vi "svx_Add SVTWav Info.vi"(6 "SVT WAV info":T1, 8 "error in (no error)":errorcluster, 11 "wave file path in":path) -> (0 "error out":errorcluster, 3 "wave file path":path)   [LabVIEW 2017]
uses:
  <vilib>/addons/_NISVFA/_Shared subVIs/Controls/SVT WAV Info.ctl
  <vilib>/addons/_NISVFA/_Shared subVIs/Controls/DAQ Coupling for SVT WAV Info.ctl
  <vilib>/addons/_NISVFA/_Shared subVIs/Controls/DAQ Polarity for SVT WAV Info.ctl
  <vilib>/addons/_NISVFA/_Shared subVIs/Controls/DAQ Terminal Configuration for SVT WAV Info.ctl
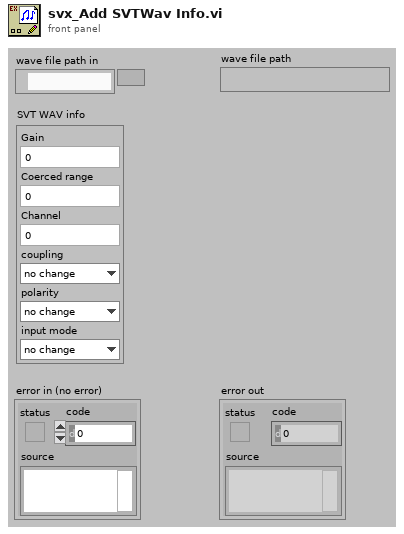
[diagram p1: front panel]
types:
  T1 = typedef "SVT WAV Info.ctl" = cluster{"Gain":u16, "Coerced range":u16, "Channel":u16, "coupling":T2, "polarity":T3, "input mode":T4}
  T2 = typedef "DAQ Coupling for SVT WAV Info.ctl" = enum16{"no change", "DC", "AC", "ground", "internal reference"}
  T3 = typedef "DAQ Polarity for SVT WAV Info.ctl" = enum16{"no change", "bipolar", "unipolar"}
  T4 = typedef "DAQ Terminal Configuration for SVT WAV Info.ctl" = enum16{"no change", "differential", "rse", "nrse", "pseudodifferential"}
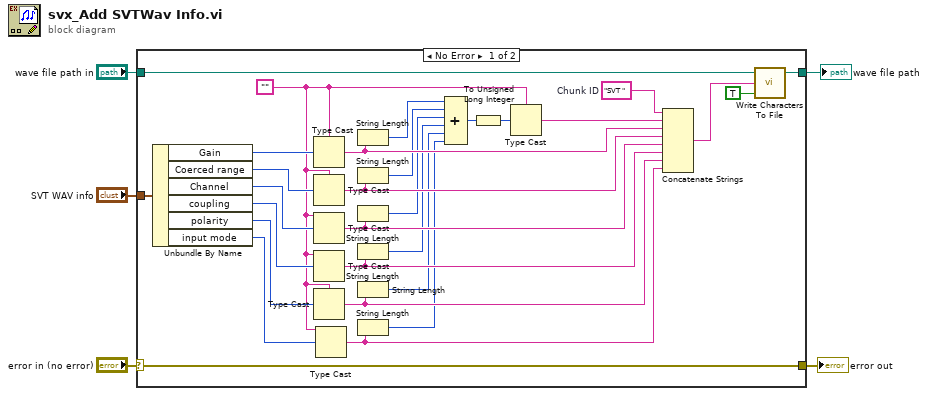
[diagram p0: block diagram]
diagram:
  n1 = case shown="No Error" "error in (no error)" {
    selector: "error in (no error)" -> [w11 w36]
    tunnel: [w11 w36] -> w4
    tunnel: "wave file path in" -> [w10 w35]
    tunnel: "SVT WAV info" -> [w9 _]
    tunnel: [w8 w35] -> w1
    frame No Error {
      w33 = "SVT "  # Chunk ID
      w12 = ""
      n2 = Unbundle By Name(w9) -> ("Gain"=w30:u16, "Coerced range"=w27:u16, "Channel"=w26:u16, "coupling"=w25:T2, "polarity"=w24:T3, "input mode"=w7:T4)
      n3 = Type Cast(type=w12, x=w30) -> (*(type *) &x=w31:string)
      n4 = Type Cast(type=w12, x=w27) -> (*(type *) &x=w23:string)
      n5 = Type Cast(type=w12, x=w26) -> (*(type *) &x=w22:string)
      n6 = Type Cast(type=w12, x=w25) -> (*(type *) &x=w21:string)
      n7 = Type Cast(type=w12, x=w24) -> (*(type *) &x=w20:string)
      n8 = Type Cast(type=w12, x=w7) -> (*(type *) &x=w6:string)
      n9 = String Length(string=w31) -> (length=w19:i32)
      n10 = String Length(string=w23) -> (length=w18:i32)
      n11 = String Length(string=w22) -> (length=w17:i32)
      n12 = String Length(string=w21) -> (length=w16:i32)
      n13 = String Length(string=w20) -> (length=w15:i32)
      n14 = String Length(string=w6) -> (length=w13:i32)
      n15 = Compound Arithmetic op=ADD(w19, w18, w17, w16, w15, w13) -> (w14:i32)
      n16 = To Unsigned Long Integer(number=w14) -> (unsigned 32bit integer=w32:u32)
      n17 = Type Cast(type=w12, x=w32) -> (*(type *) &x=w34:string)
      n18 = Concatenate Strings(w33, w34, w31, w23, w22, w21, w20, w6) -> (w28:string)
      n19 = call <vilib>:"Write Characters To File.vi"("append to file? (new file:F)"=TRUE, "character string"=w28, "file path (dialog if empty)"=w10) -> ("new file path (Not A Path if cancelled)"=w8:path)  [unwired: 2 in]
    }
    frame Error {
    }
  }
  "error out" <- w4
  "wave file path" <- w1
